vi "CompareFacesToBooleArray.vi"(8 "error in (no error)":errorcluster, 11 "CompareFaces in":refnum<k24>) -> (0 "error out":errorcluster, 2 "CompareFaces":bool[](array[boolean]), 3 "CompareFaces out":refnum<k24>)   [LabVIEW 2020, in "FaceRecognitionDotNet.lvlib" / "FaceRecognition.lvclass"]
uses:
  FaceRecognition.lvclass
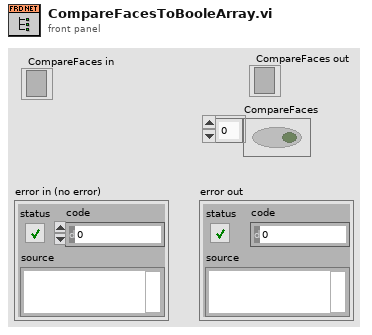
[diagram p1: front panel]
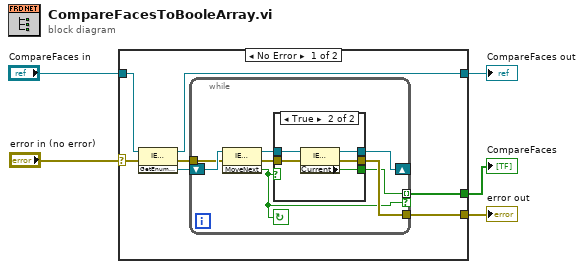
[diagram p0: block diagram]
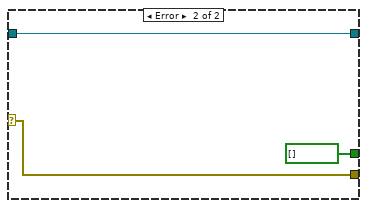
[diagram p3: hidden frame]
diagram:
  n1 = case shown="No Error" "error in (no error)" {
    selector: "error in (no error)" -> [w8 w30]
    tunnel: "CompareFaces in" -> [w12 w28]
    tunnel: [w9 w30] -> w5
    tunnel: [w7 bool[] []] -> w4
    tunnel: [w6 w28] -> w1
    frame No Error {
      n2 = invoke class="IEnumerable`1[[System.Boolean, " method="GetEnumerator"(reference=w12, error in=w8) -> (reference out=w6:refnum<k24>, error out=w10:errorcluster, "GetEnumerator"=w11:refnum<k24>)  [unwired: 1 in]
      n3 = while {
        shift-right: [w18] -> _
        shift-left: w11 -> [w20]
        tunnel: w10 -> [w17]
        tunnel: [w15] -> w9
        tunnel: [w14] -> w7 mode=indexing if=w13
        stop <- w13 continue-if-true
        n4 = invoke class="IEnumerator`1[[System.Boolean, " method="MoveNext"(reference=w20, error in=w17) -> (reference out=w19:refnum<k24>, error out=w16:errorcluster, "MoveNext"=w13:bool)  [unwired: 1 in]
        n5 = case shown="True" w13 {
          tunnel: w19 -> [w22 w27]
          tunnel: [w22 w26] -> w18
          tunnel: w16 -> [w21 w25]
          tunnel: [w21 w24] -> w15
          tunnel: [_ w23] -> w14
          frame False {
          }
          frame True {
            n6 = property class="IEnumerator`1[[System.Boolean, "(reference=w27, error in=w25) -> (reference out=w26:refnum<k24>, error out=w24:errorcluster, "Current"=w23:bool)
          }
        }
      }
    }
    frame Error {
    }
  }
  "error out" <- w5
  "CompareFaces" <- w4
  "CompareFaces out" <- w1
